vi "niRFSysCalReader Fetch Offset Error.vi"(8 "error in":errorcluster, 9 "Level (dBm)":dbl, 10 "Frequency (Hz)":dbl, 11 "niRFSysCalReader Handle":T1) -> (0 "error out":errorcluster, 2 "Error (dB)":dbl, 3 "niRFSysCalReader Handle out":T1)   [LabVIEW 2016, in "niRFSysCalReader.lvlib"]
doc: "Returns the offset error, when the source / receiver offset for the specified frequency and power / ref level is applied to the instrument.\n\n<b>Note:</b>\nOffset Error = Desired Power - Measured Power, for a TX Path\nOffset Error = Actual Power (@ Ref Plane) - Measured Power, for a RX Path"
uses:
  niRFSysCalReader.lvlib
  INCLUDES/niRFSysCalReader Handle.ctl
  INCLUDES/niRFSysCalReader Core States.ctl
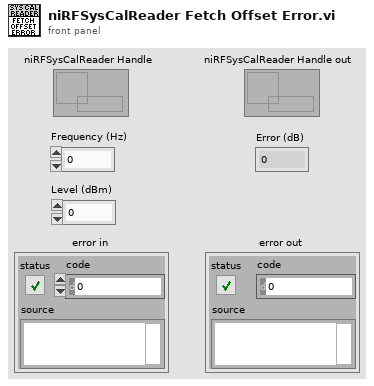
[diagram p1: front panel]
types:
  T1 = typedef "niRFSysCalReader.lvlib/niRFSysCalReader Handle.ctl" = refnum<data-value>
  T2 = typedef "niRFSysCalReader.lvlib/niRFSysCalReader Core States.ctl" = enum16{"Initialize", "Interpolator State", "Add CalData", "Get CalData", "Remove Pathloss", "Close"}
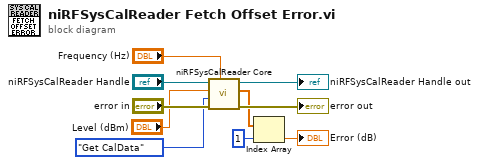
[diagram p0: block diagram]
diagram:
  n1 = call "niRFSysCalReader Core.vi"("Frequency (Hz)"="Frequency (Hz)", "error in"="error in", "niRFSysCalReader State"=niRFSysCalReader_Core_States."Get CalData" ("Cal Storage"), "Power (dBm)"="Level (dBm)", "niRFSysCalReader Handle"="niRFSysCalReader Handle") -> ("error out"=→"error out":errorcluster, "CalData Out"=w2:dbl[], "niRFSysCalReader Handle out"=→"niRFSysCalReader Handle out":T1)  [unwired: 4 in]
  n2 = Index Array(array=w2, index=1) -> (element=→"Error (dB)":dbl)
